vi "CFTS-Merge NonEPL Ouputs.vi"(0 "endpoints in":T1[](array[typedef]), 5 "NonEPL":string[](array[string])) -> (4 "endpoints out":T1[](array[typedef]))   [LabVIEW 2020]
uses:
  epl-vi-lib/Connection VIs/Typedefs/CM-Endpoint.ctl
  1056e70c-6b8a-4cee-b86c-8337879167cf.vi
  <vilib>/Comparison/Equal/Equal Functor/Equal Functor.lvclass
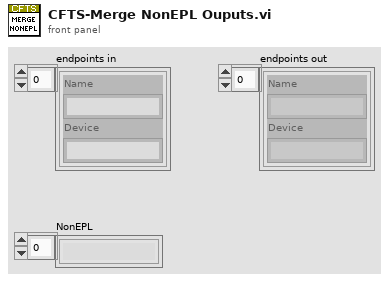
[diagram p1: front panel]
types:
  T1 = typedef "CM-Endpoint.ctl" = cluster{"Name":string, "Device":string}
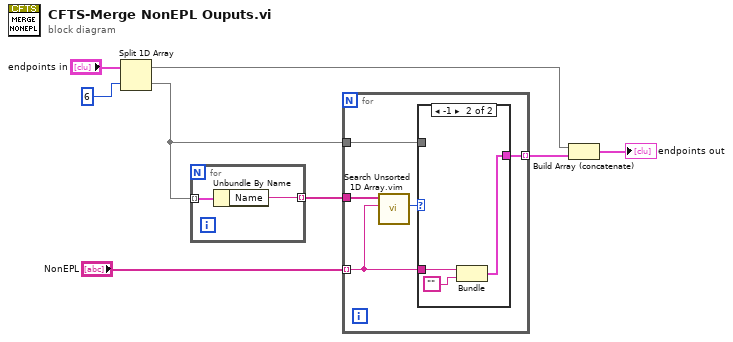
[diagram p0: block diagram]
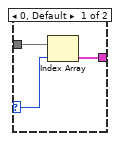
[diagram p2: hidden frame]
diagram:
  n1 = Split 1D Array(array="endpoints in", index=6 ("length")) -> (first subarray=w3:T1[], second subarray=w2:T1[])
  n2 = for {
    tunnel: w2 -> [w10] mode=indexing
    tunnel: [w9] -> w7 mode=indexing
    n3 = Unbundle By Name(w10) -> ("Name"=w9:string)
  }
  n4 = for {
    tunnel: "NonEPL" -> [w13] mode=indexing
    tunnel: w7 -> [w15]
    tunnel: w2 -> [w12]
    tunnel: [w11] -> w1 mode=indexing
    n5 = call "Search Unsorted 1D Array.vim"("element"=w13, "unsorted 1D array"=w15) -> ("index of element"=w14:i32)  [unwired: 9 in]
    n6 = case shown="-1" w14 {
      selector: w14 -> [w17 _]
      tunnel: w13 -> [_ w20]
      tunnel: w12 -> [w18 _]
      tunnel: [w16 w19] -> w11
      frame 0, Default {
        n7 = Index Array(array=w18, index=w17) -> (element=w16:T1)
      }
      frame -1 {
        n8 = Bundle("String"=w20, "") -> (w19:cluster{"String":string, string})  [unwired: 1 in]
      }
    }
  }
  n9 = Build Array (concatenate)(w3, w1) -> (→"endpoints out":T1[])
